vi "Trigger Send File.vi"() -> ()   [LabVIEW 2018]
uses:
  <vilib>/Skyline/Message/AMQP/sync/Open (Sync).vi
  <vilib>/Skyline/Message/AMQP/NI Skyline Message AMQP (Sync).lvclass
  <vilib>/Skyline/Message/NI Skyline Message.lvclass
  <vilib>/httpClient/LabVIEWHTTPClient.lvlib
panel:
  out "error out":errorcluster
  in  "topic":string="send_file"
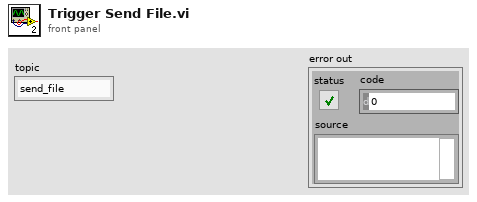
[diagram p1: front panel]
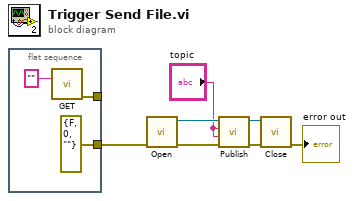
[diagram p0: block diagram]
diagram:
  n1 = flat-sequence {
    tunnel: [errorcluster {"status"=FALSE, "code"=0, "source"=""} ("error out")] -> w1
    tunnel: [w8] -> _
    frame #0 {
      n2 = call <vilib>:"GET.vi"("url"="") -> ("error out"=w8:errorcluster)  [unwired: 11 in, 3 out]
    }
  }
  n3 = call-poly <vilib>:"Open.vi"("error in (no error)"=w1) -> ("error out"=w6:errorcluster, "message sync out"=w7:refnum<class "NI Skyline Message AMQP (Sync).lvclass">)  [unwired: 9 in]
  n4 = call-dynamic "Publish.vi"("error in (no error)"=w6, "message"="topic", "topic"="topic", "message sync"=w7) -> ("error out"=w4:errorcluster, "message sync out"=w5:refnum<class "NI Skyline Message AMQP (Sync).lvclass">)  [unwired: 6 in]
  n5 = call-dynamic "Close.vi"("error in (no error)"=w4, "message sync"=w5) -> ("error out"=→"error out":errorcluster)  [unwired: 9 in]
